vi "温度曲线写入.vi"(8 "error in (no error)":errorcluster caption="错误输入（无错误）", 9 "属性值":variant[](array[variant]), 10 "属性名称":string[](array[string]), 11 "table":string="总氮") -> (0 "错误输出":errorcluster)   [LabVIEW 2016, in "斯坦道氨氮.lvlib"]
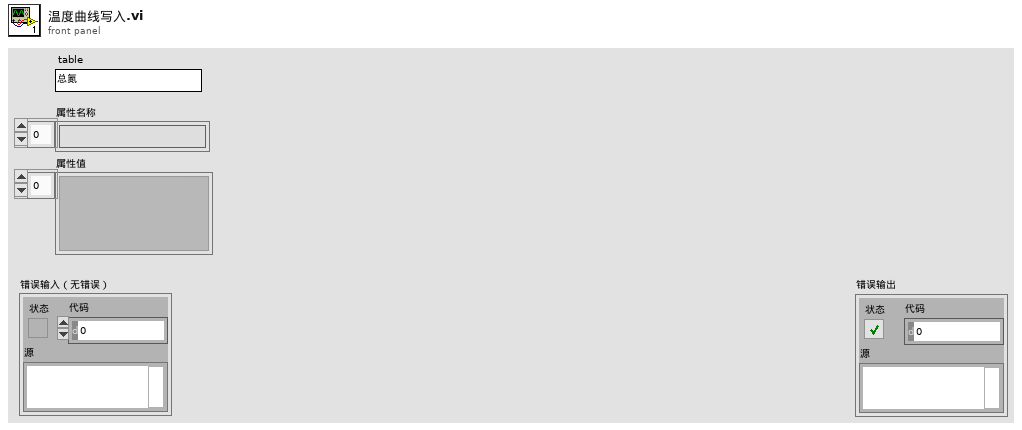
[diagram p1: front panel]
types:
  T1 = enum16{"open", "open or create", "create or replace", "create", "open (read-only)"}
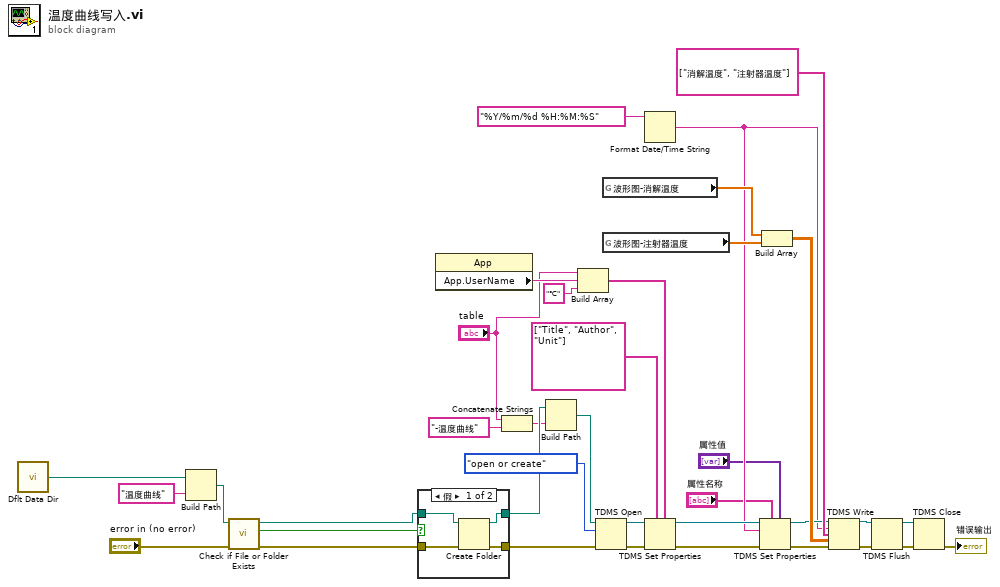
[diagram p0: block diagram]
diagram:
  n1 = call <vilib>:"Dflt Data Dir.vi"() -> ("App:Default Data Directory"=w26:path)
  n2 = Build Path(base path=w26, name or relative path="温度曲线" ("名称或相对路径")) -> (appended path=w24:path)
  n3 = call <vilib>:"Check if File or Folder Exists.vi"("error in (no error)"="error in (no error)", "path"=w24) -> ("error out"=w21:errorcluster, "file or folder exists?"=w23:bool, "dup path"=w22:path)  [unwired: 7 in]
  n4 = case shown="假" w23 {
    tunnel: w22 -> [w41 w42]
    tunnel: [w40 w42] -> w20
    tunnel: w21 -> [w39 w43]
    tunnel: [w38 w43] -> w7
    frame False {
      n5 = Create Folder(path (use dialog)=w41, error in=w39) -> (created path=w40:path, error out=w38:errorcluster)  [unwired: 1 in, 1 out]
    }
    frame True {
    }
  }
  n6 = property class="App"() -> ("App.UserName"=w35:string)  [unwired: 2 in, 2 out]
  n7 = Concatenate Strings("table", "-温度曲线" ("字符串")) -> (w18:string)
  n8 = Build Path(base path=w20, name or relative path=w18) -> (appended path=w17:path)
  n9 = Build Array("table", w35, "℃" ("元素")) -> (w33:string[])
  n10 = TDMS Open(8:w7, 10:T1."open or create" ("操作(0:open)"), 11:w17) -> (0:w36:errorcluster, 3:w37:refnum<k34>)  [unwired: 4 in]
  n11 = global read "VAR总磷总氮全局变量.vi" "波形图-消解温度"() -> (w28:dbl[])
  n12 = global read "VAR总磷总氮全局变量.vi" "波形图-注射器温度"() -> (w27:dbl[])
  n13 = Format Date/Time String(time format string (%c)="%Y/%m/%d %H:%M:%S" ("时间格式字符串(%c)")) -> (date/time string=w11:string)  [unwired: 2 in]
  n14 = TDMS Set Properties(5:w33, 7:string[] ["Title", "Author", "Unit"] ("property names"), 8:w36, 11:w37) -> (0:w15:errorcluster, 3:w13:refnum<k34>)  [unwired: 2 in, 2 out]
  n15 = TDMS Set Properties(5:"属性值", 7:"属性名称", 8:w15, 10:w11, 11:w13) -> (0:w14:errorcluster, 3:w12:refnum<k34>)  [unwired: 1 in, 2 out]
  n16 = Build Array(w28, w27) -> (w31:dbl[][])
  n17 = TDMS Write(0:w12, 5:w11, 7:string[] ["消解温度", "注射器温度"] ("通道名输入（无标题）"), 9:w31, 11:w14) -> (4:w4:refnum<k34>, 15:w3:errorcluster)  [unwired: 1 in, 2 out]
  n18 = TDMS Flush(4:w3, 7:w4) -> (0:w2:errorcluster, 3:w1:refnum<k34>)
  n19 = TDMS Close(8:w2, 11:w1) -> (0:→"错误输出":errorcluster)  [unwired: 1 out]
